vi "Read Job Report.vi"(8 "error in (no error)":errorcluster, 11 "JobReport in":refnum<class "JobReport.lvclass">) -> (0 "error out":errorcluster, 2 "Job Report":T1, 3 "JobReport out":refnum<class "JobReport.lvclass">)   [LabVIEW 2013, in "openCronJob.lvlib" / "JobReport.lvclass"]
uses:
  JobReport.lvclass
  Job/Job Report -- cluster.ctl
  JobReport.lvclass/JobReport.ctl
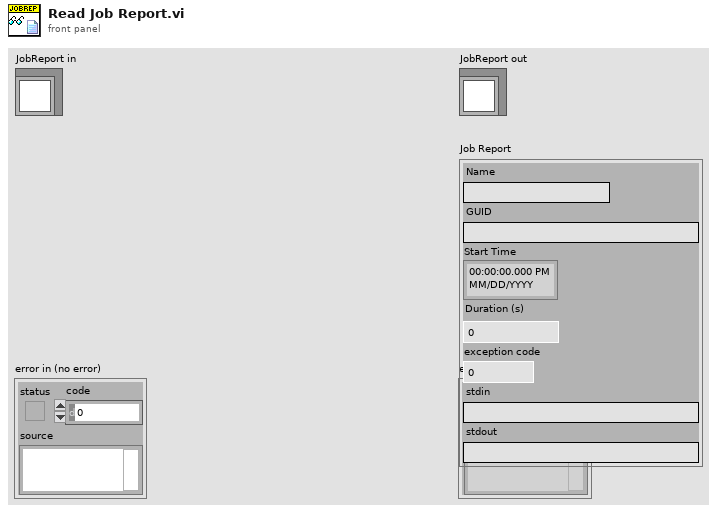
[diagram p1: front panel]
types:
  T1 = typedef "openCronJob.lvlib/JobReport.lvclass/Job Report -- cluster.ctl" = cluster{"Name":string, "GUID":string, "Start Time":timestamp, "Duration (s)":dbl, "exception code":i32, "stdin":string, "stdout":string}
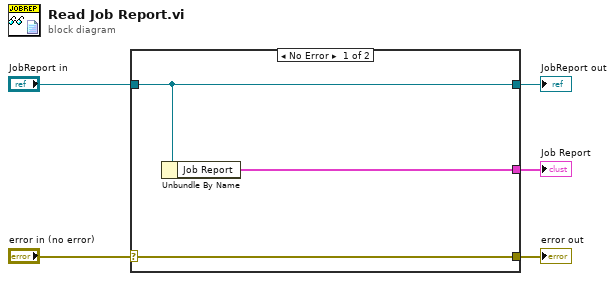
[diagram p0: block diagram]
diagram:
  n1 = case shown="No Error" "error in (no error)" {
    selector: "error in (no error)" -> [w8 w9]
    tunnel: [w8 w9] -> w4
    tunnel: [w7 w10] -> w2
    tunnel: "JobReport in" -> [w7 w10]
    tunnel: [w6 _] -> w1
    frame No Error {
      n2 = Unbundle By Name(w7) -> ("Job Report"=w6:T1)
    }
    frame Error {
    }
  }
  "error out" <- w4
  "JobReport out" <- w2
  "Job Report" <- w1
